vi "GetFullPath.vi"(0 "string Path in":string) -> (1 "Path is Ok?":bool, 2 "absolute path":path)   [LabVIEW 2010]
panel:
  out "error out":errorcluster
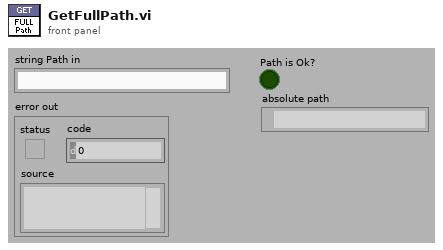
[diagram p1: front panel]
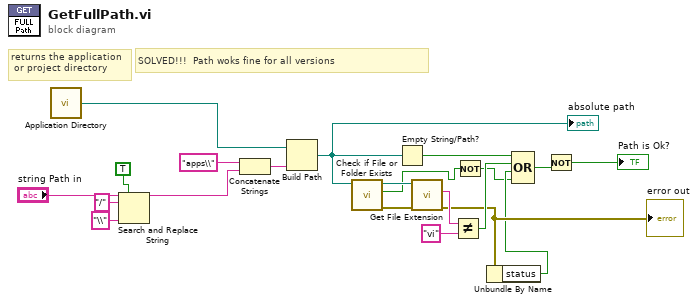
[diagram p0: block diagram]
diagram:
  # "returns the application\n or project directory"
  # "SOLVED!!!  Path woks fine for all versions"
  n1 = call <vilib>:"Application Directory.vi"() -> ("Application Directory"=w5:path)
  n2 = Search and Replace String(replace all?=TRUE ("replace all? (F)"), input string="string Path in", search string="/", replace string="\\" ("replace string (\"\")")) -> (result string=w9:string)  [unwired: 1 in, 6 out]
  n3 = Concatenate Strings("apps\\" ("string"), w9) -> (w21:string)
  n4 = Build Path(base path=w5, name or relative path=w21) -> (appended path=w14:path)
  "absolute path" <- w14
  n5 = call <vilib>:"Check if File or Folder Exists.vi"("path"=w14) -> ("error out"=w18:errorcluster, "file or folder exists?"=w2:bool, "dup path"=w19:path)  [unwired: 1 in, 7 out]
  n6 = Empty String/Path?(string/path=w14) -> (empty?=w16:bool)
  n7 = call <vilib>:"Get File Extension.vi"("error in (no error)"=w18, "file"=w19) -> ("error out"=w4:errorcluster, "lowercase file extension"=w6:string)  [unwired: 8 out]
  "error out" <- w4
  n8 = Not Equal?(x=w6, y="vi") -> (x != y?=w15:bool)
  n9 = Not(x=w2) -> (.not. x?=w1:bool)
  n10 = Unbundle By Name(w4) -> ("status"=w3:bool)
  n11 = Compound Arithmetic op=OR(w16, w15, w3, w1) -> (w8:bool)
  n12 = Not(x=w8) -> (.not. x?=→"Path is Ok?":bool)
